vi "CheckCoordinates.vi"(0 "reference in":refnum<class "Map.lvclass">, 1 "X":i32, 2 "Y":i32, 5 "error in (no error)":errorcluster) -> (14 "reference out":refnum<class "Map.lvclass">, 15 "SurfaceType":T1, 19 "error out":errorcluster)   [LabVIEW 2019, in "Map.lvclass"]
doc: "Checks is position is a empty or contains a wall"
uses:
  Map.lvclass
  SurfaceType.ctl
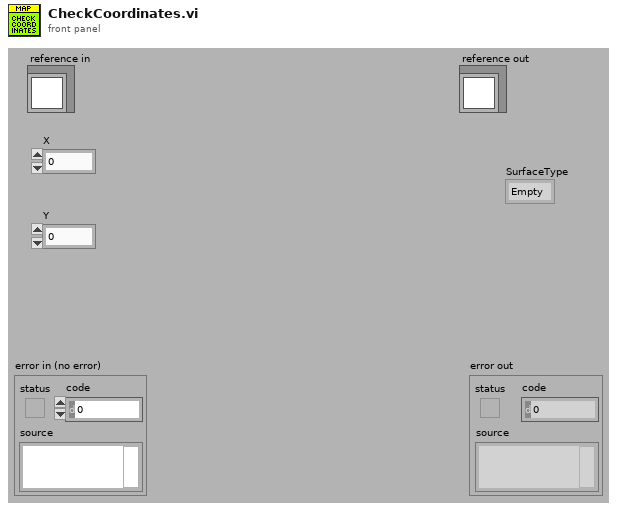
[diagram p1: front panel]
types:
  T1 = typedef "Map.lvclass/SurfaceType.ctl" = enum16{"Empty", "Wall"}
  T2 = typedef "Map.lvclass/ObjectAttributes.ctl" = cluster{"Width":i32, "Height":i32, "Map":bool[][]}
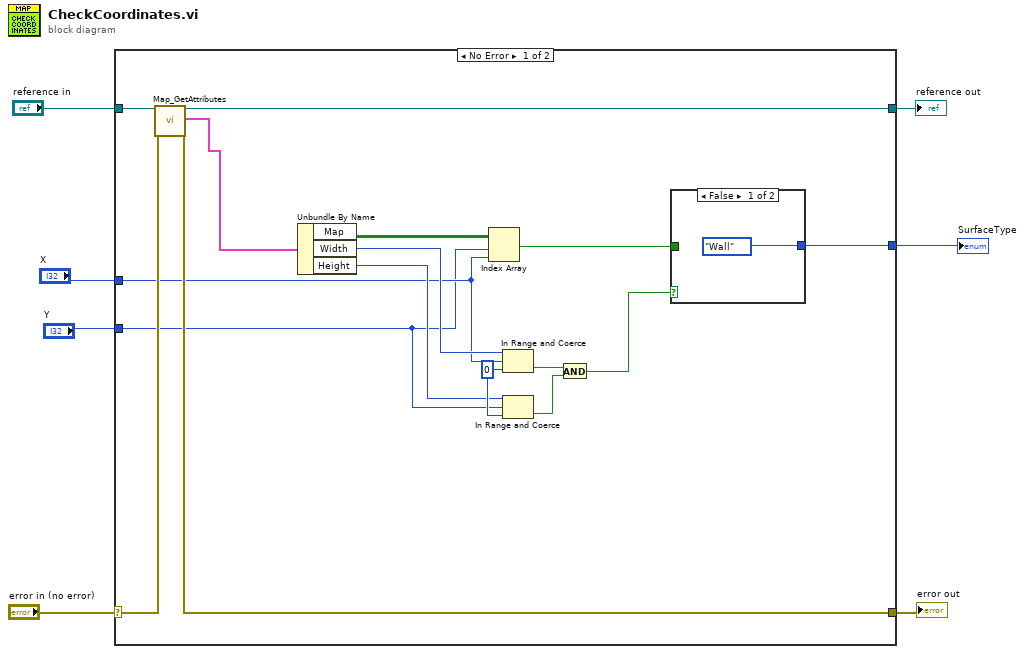
[diagram p0: block diagram]
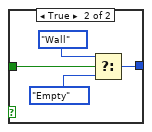
[diagram p2: hidden frame]
diagram:
  n1 = case shown="No Error" "error in (no error)" {
    selector: "error in (no error)" -> [w23 w30]
    tunnel: [w22 w30] -> w6
    tunnel: [w20 w29] -> w4
    tunnel: "reference in" -> [w21 w29]
    tunnel: [w11 _] -> w3
    tunnel: "X" -> [w9 _]
    tunnel: "Y" -> [w8 _]
    frame No Error {
      w16 = 0 ("lower limit")
      n2 = call "Map_GetAttributes.vi"("reference in"=w21, "error in (no error)"=w23) -> ("reference out"=w20:refnum<class "Map.lvclass">, "Attributes"=w10:T2, "error out"=w22:errorcluster)  [unwired: 15 out]
      n3 = Unbundle By Name(w10) -> ("Map"=w19:bool[][], "Width"=w17:i32, "Height"=w15:i32)
      n4 = Index Array(array=w19, index (row)=w8, index (col)=w9) -> (element=w18:bool)
      n5 = In Range and Coerce(upper limit=w17, x=w9, lower limit=w16) -> (In Range?=w14:bool)  [unwired: 1 out]
      n6 = In Range and Coerce(upper limit=w15, x=w8, lower limit=w16) -> (In Range?=w13:bool)  [unwired: 1 out]
      n7 = And(x=w14, y=w13) -> (x .and. y?=w12:bool)
      n8 = case shown="False" w12 {
        tunnel: w18 -> [_ w28]
        tunnel: [SurfaceType."Wall" ("SurfaceType") w27] -> w11
        frame False {
        }
        frame True {
          n9 = Select(t=SurfaceType."Wall" ("SurfaceType"), s=w28, f=SurfaceType."Empty" ("SurfaceType")) -> (s? t:f=w27:T1)
        }
      }
    }
    frame Error {
    }
  }
  "error out" <- w6
  "reference out" <- w4
  "SurfaceType" <- w3
